vi "Go to Lift Height.vi"(8 "Time to Settle":u32=500, 11 "Lift Height to Go To":T1(ring)=enum."Hatch Panel Zone 3") -> ()   [LabVIEW 2018]
uses:
  SubSystems/Lift/Lift Global.vi
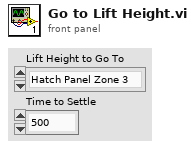
[diagram p1: front panel]
types:
  T1 = enum16{"Hatch Panel Zone 1", "Hatch Panel Zone 2", "Hatch Panel Zone 3", "Cargo Zone 1", "Cargo Zone 2", "Cargo Zone 3", "Cargo Ship Zone"}
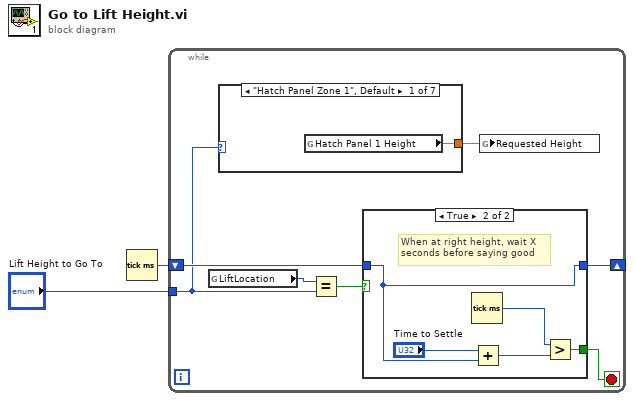
[diagram p0: block diagram]
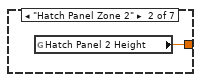
[diagram p2: hidden frame]
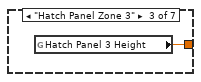
[diagram p3: hidden frame]
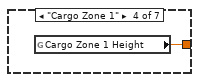
[diagram p4: hidden frame]
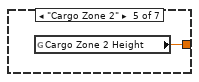
[diagram p5: hidden frame]
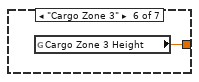
[diagram p6: hidden frame]
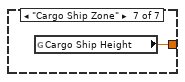
[diagram p7: hidden frame]
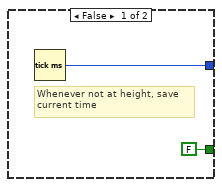
[diagram p8: hidden frame]
diagram:
  n1 = Tick Count (ms)() -> (millisecond timer value=w1:u32)
  n2 = while {
    tunnel: "Lift Height to Go To" -> [w3]
    shift-right: [w6] -> _
    shift-left: w1 -> [w8]
    stop <- w5 stop-if-true
    n3 = global read "Lift Global.vi" "LiftLocation"() -> (w9:T1)
    n4 = case shown="\"Hatch Panel Zone 1\", Default" w3 {
      tunnel: [w10 w11 w12 w13 w14 w15 w16] -> w4
      frame "Hatch Panel Zone 1", Default {
        n5 = global read "Lift Global.vi" "Hatch Panel 1 Height"() -> (w10:dbl)
      }
      frame "Hatch Panel Zone 2" {
        n6 = global read "Lift Global.vi" "Hatch Panel 2 Height"() -> (w11:dbl)
      }
      frame "Hatch Panel Zone 3" {
        n7 = global read "Lift Global.vi" "Hatch Panel 3 Height"() -> (w12:dbl)
      }
      frame "Cargo Zone 1" {
        n8 = global read "Lift Global.vi" "Cargo Zone 1 Height"() -> (w13:dbl)
      }
      frame "Cargo Zone 2" {
        n9 = global read "Lift Global.vi" "Cargo Zone 2 Height"() -> (w14:dbl)
      }
      frame "Cargo Zone 3" {
        n10 = global read "Lift Global.vi" "Cargo Zone 3 Height"() -> (w15:dbl)
      }
      frame "Cargo Ship Zone" {
        n11 = global read "Lift Global.vi" "Cargo Ship Height"() -> (w16:dbl)
      }
    }
    n12 = Equal?(x=w9, y=w3) -> (x = y?=w7:bool)
    n13 = case shown="True" w7 {
      tunnel: w8 -> [_ w23]
      tunnel: [w18 w23] -> w6
      tunnel: [FALSE w19] -> w5
      frame False {
        # "Whenever not at height, save \ncurrent time"
        n14 = Tick Count (ms)() -> (millisecond timer value=w18:u32)
      }
      frame True {
        # "When at right height, wait X\nseconds before saying good"
        n15 = Tick Count (ms)() -> (millisecond timer value=w21:u32)
        n16 = Add(x="Time to Settle", y=w23) -> (x+y=w20:u32)
        n17 = Greater?(x=w21, y=w20) -> (0:w19:bool)
      }
    }
    n18 = global write "Lift Global.vi" "Requested Height"(w4) -> ()
  }
